vi "searchShopInfo.vi"(2 "商店信息out":cluster{"店名":string, "营业":bool, "位置":string}, 3 "Tree引用句柄 2":refnum<vi>, 8 "error in (no error)":errorcluster caption="错误输入（无错误）", 10 "商店信息":cluster{"店名":string, "营业":bool, "位置":string}, 11 "Tree引用句柄":refnum<vi>) -> (0 "error out":errorcluster caption="错误输出")   [LabVIEW 2013, in "ShopBase.lvclass"]
doc: "该模板用于创建子VI。"
uses:
  ShopBase.lvclass
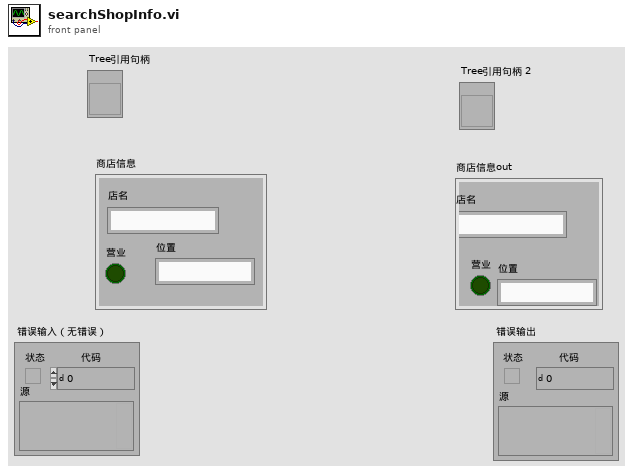
[diagram p1: front panel]
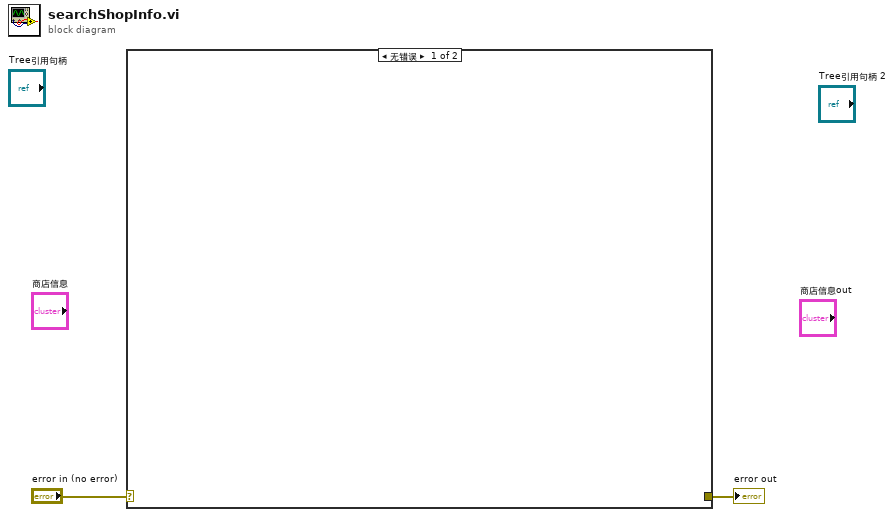
[diagram p0: block diagram]
diagram:
  n1 = case shown="无错误" "error in (no error)" {
    selector: "error in (no error)" -> [_ w3]
    tunnel: [_ w3] -> w1
    frame No Error {
    }
    frame Error {
    }
  }
  "error out" <- w1
